vi "Lab5_PSK1.vi"() -> ()   [LabVIEW 2019]
uses:
  <vilib>/addons/Modulation/Digital/General/MT Generate Bits (Galois, PN Order).vi
  <vilib>/addons/Modulation/Digital/Support/Common/Validators/mod_Generate Bits Validate.vi
  <vilib>/addons/Modulation/Analog/support/mod_Set Error Source.vi
  <vilib>/addons/Modulation/Digital/Support/Common/Validators/mod_AWGN Validate.vi
  <vilib>/addons/Modulation/Digital/Impairments/subVIs/mod_createSeeds.vi
  <vilib>/addons/Modulation/Digital/Support/Common/Validators/mod_Validate Samples Per Symbol.vi
  <vilib>/addons/Modulation/Analog/support/Validators/mod_Validate Complex Waveform.vi
  <vilib>/addons/Modulation/Analog/support/Validators/mod_WFErrorHandler.vi
  <vilib>/addons/Modulation/Digital/General/MT Generate PSK System Parameters(M).vi
  <vilib>/addons/Modulation/Digital/General/subVIs/mod_Generate Bits PN Sequence.vi
  <vilib>/addons/Modulation/Digital/Support/Common/Validators/mod_Generate Filter Coefficients Validate.vi
  <vilib>/addons/Modulation/Digital/General/subVIs/mod_Generate Filter Coefficients.vi
  <vilib>/Analysis/1siggen.llb/Gaussian White Noise (obs 90).vi
  <vilib>/addons/Modulation/Digital/General/MT Format Eye Diagram (complex).vi
  <vilib>/addons/Modulation/niDMT.lvlib
panel:
  in  "pulse shaping filter":u16(ring) items=["none", "Raised Cosine", "Root Raised Cos", "Gaussian"]
  out "Cannel Input(Baseband)":cluster{"t0":dbl, "dt":dbl, "Y":dbl[]}(graph)
  out "Cannel Output(Baseband)":cluster{"t0":dbl, "dt":dbl, "Y":dbl[]}(graph)
  in  "Eb/N0 (dB)":dbl=10.0 format="%.2f"
  in  "M-PSK":i32(ring)=4 items=["2"=2, "4"=4, "8"=8, "16"=16]
  in  "Tab Control":enum32{"Constelllation", "Eye Diagram"}(tab)
  out "Constellation Plot":T1(graph)
  out "Eye Diagram":cluster{"t0":dbl, "dt":dbl, "Y":dbl[]}[](graph)
  in  "Reset":bool=TRUE
  in  "stop":bool
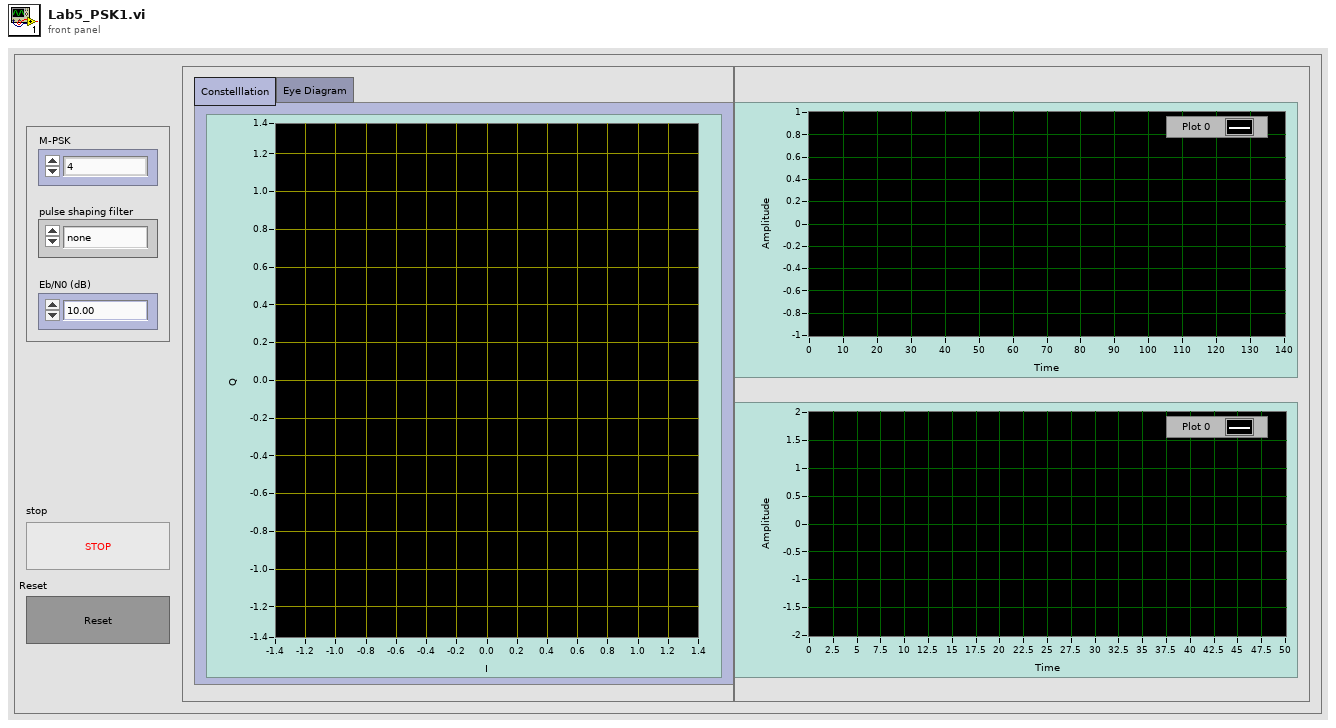
[diagram p1: front panel]
types:
  T1 = cluster{"Decimated Array":dbl[], "Decimated Array":dbl[]}[]
  T2 = enum16{"FSK", "PSK", "QAM", "MSK", "PAM", "ASK", "CPM"}
  T3 = cluster{"samples per symbol (16)":i32, "symbol map":cdb[], "differential PSK":enum16{"disable", "enable"}, "PSK type":u16}
  T4 = typedef "niAMT.lvlib/Complex Data Waveform.ctl" = cluster{"t0":dbl, "dt":dbl, "Y":cdb[]}
  T5 = cluster{"constellation":dbl[], "oversampled data":dbl[]}[]
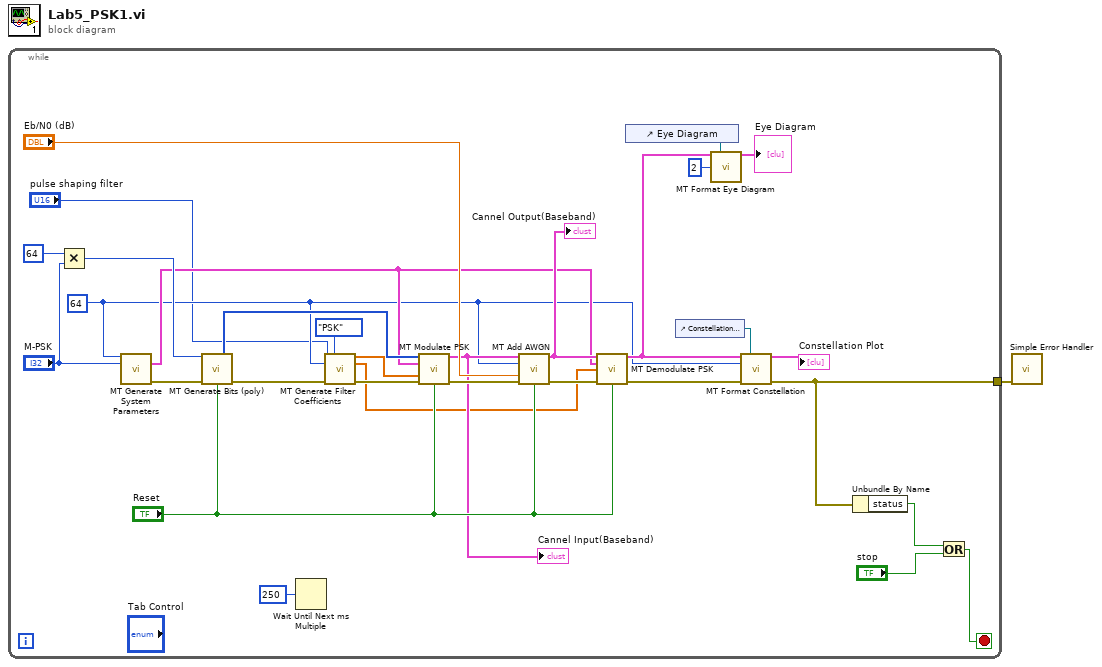
[diagram p0: block diagram]
diagram:
  n1 = while {
    tunnel: [w8] -> w1
    stop <- w24 stop-if-true
    w3 = 64 ("samples per symbol (16)")
    n2 = Multiply(x=64, y="M-PSK") -> (x*y=w20:i32)
    n3 = call-poly <vilib>:"MT Generate System Parameters.vi"("samples per symbol (16)"=w3, "M-PSK (4)"="M-PSK") -> ("PSK system parameters"=w14:T3, "error out"=w29:errorcluster)  [unwired: 11 in, 1 out]
    n4 = call-poly <vilib>:"MT Generate Bits (poly).vi"("total bits (128)"=w20, "error in (no error)"=w29, "reset? (T)"="Reset") -> ("output bit stream"=w30:i8[], "error out"=w28:errorcluster)  [unwired: 10 in, 1 out]
    n5 = Wait Until Next ms Multiple(millisecond multiple=u32 250) -> ()  [unwired: 1 out]
    n6 = call <vilib>:"MT Generate Filter Coefficients.vi"("pulse shaping filter (none)"="pulse shaping filter", "modulation type"=T2."PSK", "pulse shaping samples per symbol (16)"=w3, "error in (no error)"=w28) -> ("pulse shaping filter coefficients"=w16:dbl[], "matched filter coefficients"=w15:dbl[], "error out"=w27:errorcluster)  [unwired: 9 in]
    n7 = call <vilib>:"MT Modulate PSK.vi"("input bit stream"=w30, "PSK system parameters"=w14, "pulse shaping filter coefficients"=w16, "error in (no error)"=w27, "reset? (T)"="Reset") -> ("output complex waveform"=w18:T4, "error out"=w26:errorcluster)  [unwired: 8 in, 1 out]
    "Cannel Input(Baseband)" <- w18
    n8 = call <vilib>:"MT Add AWGN.vi"("input complex waveform"=w18, "samples per symbol (16)"=w3, "Eb/N0 (10 dB)"="Eb/N0 (dB)", "error in (no error)"=w26, "reset? (T)"="Reset") -> ("output complex waveform"=w17:T4, "error out"=w25:errorcluster)  [unwired: 8 in, 1 out]
    "Cannel Output(Baseband)" <- w17
    n9 = call <vilib>:"MT Demodulate PSK.vi"("input complex waveform"=w17, "PSK system parameters"=w14, "matched filter coefficients"=w15, "error in (no error)"=w25, "reset? (T)"="Reset") -> ("recovered complex waveform"=w7:T4, "error out"=w9:errorcluster)  [unwired: 6 in, 3 out]
    n10 = control-ref of="Eye Diagram"() -> (w10:refnum<vi>)
    n11 = control-ref of="Constellation Plot"() -> (w12:refnum<vi>)
    n12 = call-poly <vilib>:"MT Format Eye Diagram.vi"("waveform"=w7, "eye diagram reference"=w10, "eye length"=2) -> ("eye diagram"=→"Eye Diagram":cluster{"t0":dbl, "dt":dbl, "Y":dbl[]}[])  [unwired: 4 in, 8 out]
    n13 = call <vilib>:"MT Format Constellation.vi"("waveform"=w7, "constellation reference"=w12, "samples per symbol"=w3, "error in (no error)"=w9) -> ("constellation graph"=→"Constellation Plot":T5, "error out"=w8:errorcluster)  [unwired: 1 in, 9 out]
    n14 = Unbundle By Name(w8) -> ("status"=w5:bool)
    n15 = Or(x=w5, y="stop") -> (x .or. y?=w24:bool)
  }
  n16 = call <vilib>:"Simple Error Handler.vi"("error in (no error)"=w1) -> ()  [unwired: 4 in, 5 out]
